vi "MaxXY.vi"(1 "input_xyz_um":T2, 2 "parameters_xy_scan":T1={"image_size_xy_um"=1.0, "frame_size_xy_px"=10, "pixel_dwell_ms"=1.0} {"pixel_dwell_ms" format="%#_13g"; "image_size_xy_um" format="%#_13g"}) -> (6 "mse":cluster{"mse_y":dbl, "mse_x":dbl}, 7 "output_xyz_um":T2, 8 "BestGaussianFit":cluster{dbl[], dbl[]}, 9 "SumXY":cluster{dbl[], dbl[]}, 10 "image":dbl[][](graph))   [LabVIEW 2018]
uses:
  <vilib>/Analysis/1siggen.llb/Ramp Pattern by Samples.vi
  <vilib>/Analysis/NI_AALPro.lvlib
  <vilib>/Analysis/NI_AALBase.lvlib
panel:
  out "section_y":dbl[][](graph)
  out "section_x":dbl[][](graph)
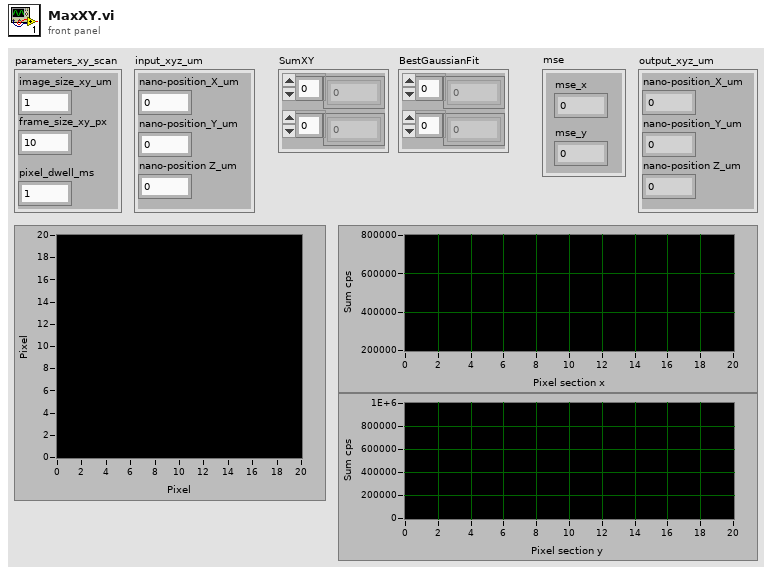
[diagram p1: front panel]
types:
  T1 = cluster{"image_size_xy_um":dbl, "frame_size_xy_px":u32, "pixel_dwell_ms":dbl}
  T2 = cluster{"nano-position_X_um":sgl, "nano-position_Y_um":sgl, "nano-position Z_um":sgl}
  T3 = cluster{"Best Gaussian Fit":dbl[], "Best Gaussian Fit":dbl[]}
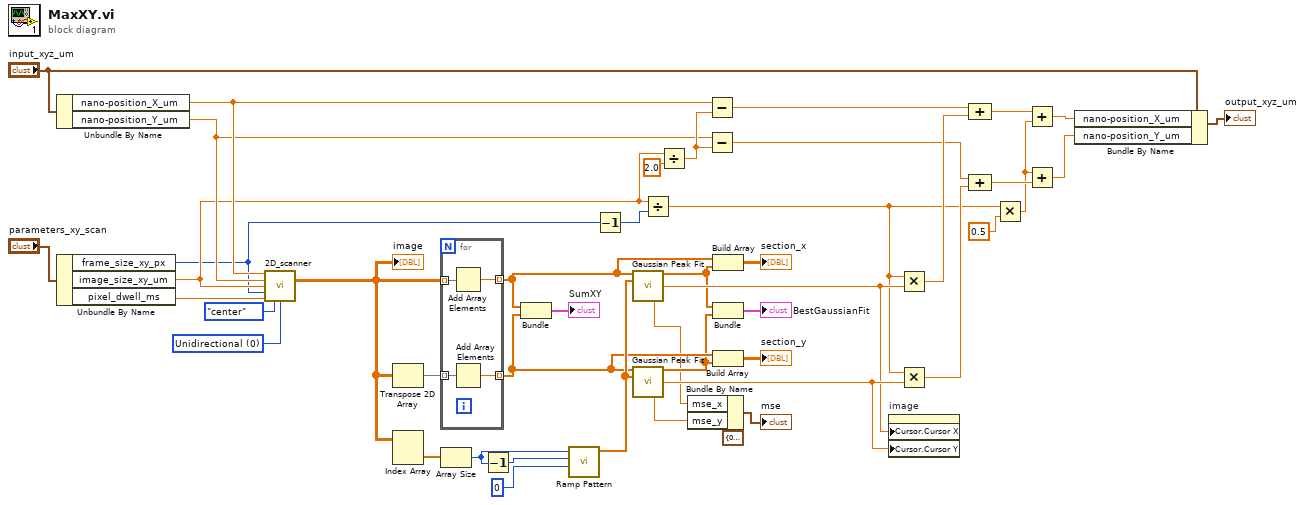
[diagram p0: block diagram]
diagram:
  w5 = u32 0 items=["Unidirectional", "Bidirectional"]
  n1 = Unbundle By Name("input_xyz_um") -> ("nano-position_X_um"=w26:sgl, "nano-position_Y_um"=w25:sgl)
  n2 = Unbundle By Name("parameters_xy_scan") -> ("frame_size_xy_px"=w23:u32, "image_size_xy_um"=w24:dbl, "pixel_dwell_ms"=w22:dbl)
  n3 = call "2D_scanner.vi"("pos-start_x"=w26, "pos-start_y"=w25, "image_size_x_um"=w24, "frame_size_x_px"=w23, "pixel_dwell_ms"=w22, "pos_start"=enum32{"bottom-left", "center"}."center", "scan_direction"=w5) -> ("image_out"=w20:dbl[][])  [unwired: 8 in]
  "image" <- w20
  n4 = Transpose 2D Array(2D array=w20) -> (transposed array=w19:dbl[][])
  n5 = Index Array(array=w20) -> (element=w18:dbl[])  [unwired: 2 in]
  n6 = for {
    tunnel: w20 -> [w49] mode=indexing
    tunnel: w19 -> [w48] mode=indexing
    tunnel: [w47] -> w8 mode=indexing
    tunnel: [w46] -> w10 mode=indexing
    n7 = Add Array Elements(numeric array=w49) -> (sum=w47:dbl)
    n8 = Add Array Elements(numeric array=w48) -> (sum=w46:dbl)
  }
  n9 = Array Size(array=w18) -> (size(s)=w17:i32)
  n10 = Decrement(x=w17) -> (x-1=w16:i32)
  n11 = Bundle(w8, w10) -> (→"SumXY":cluster{dbl[], dbl[]})  [unwired: 1 in]
  n12 = call-poly <vilib>:"Ramp Pattern.vi"("start"=u32 0, "end"=w16, "samples"=w17) -> ("Ramp Pattern"=w14:dbl[])  [unwired: 7 in, 1 out]
  n13 = Decrement(x=w23) -> (x-1=w39:u32)
  n14 = call <vilib>:"Gaussian Peak Fit.vi"("Y"=w8, "X"=w14) -> ("Best Gaussian Fit"=w7:dbl[], "center"=w37:dbl, "residue"=w2:dbl)  [unwired: 7 in, 4 out]
  n15 = call <vilib>:"Gaussian Peak Fit.vi"("Y"=w10, "X"=w14) -> ("Best Gaussian Fit"=w6:dbl[], "center"=w38:dbl, "residue"=w3:dbl)  [unwired: 7 in, 4 out]
  n16 = Divide(x=w24, y=w39) -> (x/y=w36:dbl)
  n17 = Divide(x=w24, y=2.0) -> (x/y=w41:dbl)
  n18 = Bundle By Name(cluster=cluster{"mse_y":dbl, "mse_x":dbl} {"mse_y"=0.0, "mse_x"=0.0} ("mse"), "mse_x"=w2, "mse_y"=w3) -> (→"mse":cluster{"mse_y":dbl, "mse_x":dbl})
  n19 = Subtract(x=w26, y=w41) -> (x-y=w40:dbl)
  n20 = Subtract(x=w25, y=w41) -> (x-y=w30:dbl)
  n21 = Build Array(w8, w7) -> (→"section_x":dbl[][])
  n22 = Bundle("Best Gaussian Fit"=w7, "Best Gaussian Fit"=w6) -> (→"BestGaussianFit":T3)  [unwired: 1 in]
  n23 = Build Array(w10, w6) -> (→"section_y":dbl[][])
  n24 = property on="image" class="IntGraph (strict)"("Cursor.Cursor X"=w37, "Cursor.Cursor Y"=w38) -> ()  [unwired: 2 in, 2 out]
  n25 = Multiply(x=w36, y=w37) -> (x*y=w43:dbl)
  n26 = Multiply(x=w36, y=w38) -> (x*y=w45:dbl)
  n27 = Compound Arithmetic op=ADD(w40, w43) -> (w33:dbl)
  n28 = Compound Arithmetic op=ADD(w30, w45) -> (w44:dbl)
  n29 = Multiply(x=w36, y=0.5) -> (x*y=w34:dbl)
  n30 = Add(x=w33, y=w34) -> (x+y=w29:dbl)
  n31 = Add(x=w34, y=w44) -> (x+y=w28:dbl)
  n32 = Bundle By Name(cluster="input_xyz_um", "nano-position_X_um"=w29, "nano-position_Y_um"=w28) -> (→"output_xyz_um":T2)
